vi "GetDoorStatus.vi"(8 "error in":errorcluster, 11 "VISA resource name":refnum<visa-resource-name>) -> (0 "error out":errorcluster, 2 "Door Status":string, 3 "VISA resource name out":refnum<visa-resource-name>)   [LabVIEW 2023, in "Thermotron 8800.lvlib"]
doc: "DOOR\nCommand name: Send door status\nCommand type: System status\nDescription: This command returns 1 if there is a “Door” digital input defined and it is currently\nclosed. It returns 0 if the door is open or there is no digital input defined for it.\nSyntax: DOOR?\nData type: Integer\nQuery example: DOOR?\n8800 response: 1 (There is a “Door” digital input defined and it is currently closed.)"
uses:
  Thermotron 8800.lvlib
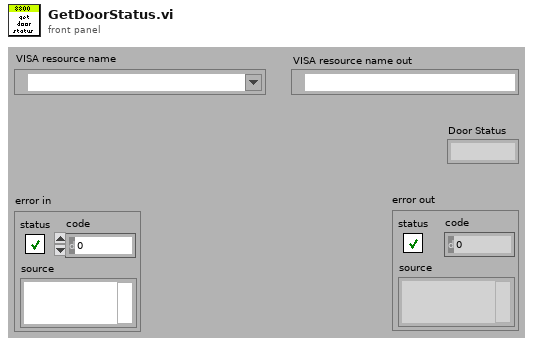
[diagram p1: front panel]
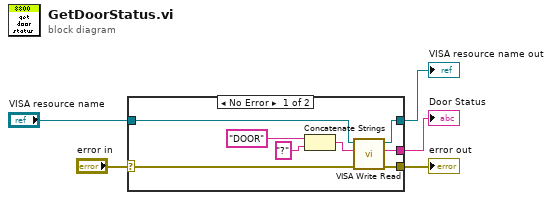
[diagram p0: block diagram]
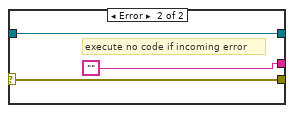
[diagram p2: hidden frame]
diagram:
  n1 = case shown="No Error" "error in" {
    selector: "error in" -> [w10 w15]
    tunnel: [w7 w15] -> w4
    tunnel: [w8 w16] -> w3
    tunnel: "VISA resource name" -> [w9 w16]
    tunnel: [w6 ""] -> w1
    frame No Error {
      n2 = Concatenate Strings("DOOR" ("8800 Command"), "?" ("8800 Command")) -> (w13:string)
      n3 = call "VISA Write Read.vi"("error in (no error)"=w10, "8800 Command"=w13, "VISA Refnum in"=w9) -> ("error out"=w7:errorcluster, "read buffer"=w6:string, "VISA Refnum out"=w8:refnum<visa-resource-name>)  [unwired: 6 in]
    }
    frame Error {
      # "execute no code if incoming error"
    }
  }
  "VISA resource name out" <- w3
  "error out" <- w4
  "Door Status" <- w1
